vi "junk48.vi"() -> ()   [LabVIEW 2018]
uses:
  <vilib>/FTP/NI_FTP.lvlib
  <vilib>/Utility/error.llb/DialogType.ctl
panel:
  out "standard output":string
  out "message":string=" INSTRUCTIONS:\r\rNormal Use:  When using subVIs that incorporate the error in/error out (or error I/O) structure, place this handler where you want to inform the user of an error, typically at the end of the I/O data path, as the last action of the program.  If the error in error? is ERROR, the handler creates a message describing the error and its source.  If the type of dialog = 1 (default), the message is displayed to the user, who can only acknowedge it.  If the type = 2, the user can acknowledge the message or abort execution; aborting a program with active I/O is not recommended.  If the type = 0, no message is displayed; this is used to process the error programmatically, and the error out cluster elements are wired to individual terminals for that reason.  \r\rOther Use:\n\r\nlocal testing.  To test the error code of a subVI or function that does not have the error I/O structure, you can wire its error code and a source string to the local error code and error source inputs.  If error in error? indicates no error and error code is not equal to 0, the local code and source are substituted for the error in values, and error? is set TRUE (ERROR)."
  out "text 2":string
  in  "file (use dialog) 2":path=path "C:/tmp/junk1.txt"
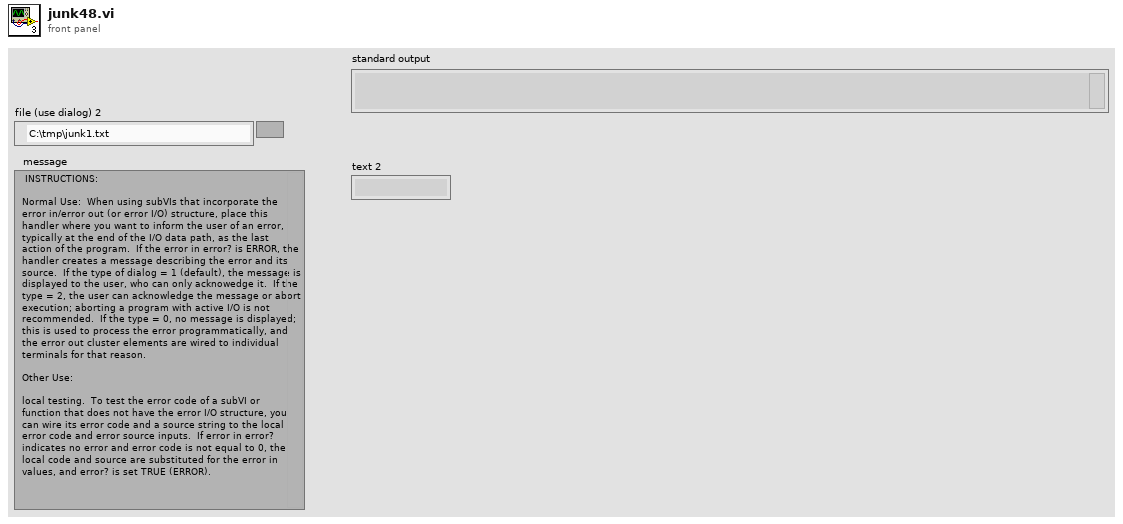
[diagram p1: front panel]
types:
  T1 = typedef "DialogType.ctl" = u16
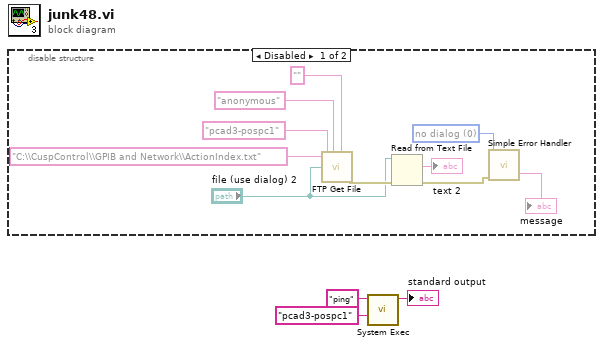
[diagram p0: block diagram]
diagram:
  n1 = disable-structure shown="Disabled" {
    frame Disabled {
      w5 = T1 0 items=["no dialog", "OK message", "continue or stop message", "OK message + warnings", "continue/stop + warnings"] ("type of dialog (OK msg:1)")
      n2 = call <vilib>:"FTP Get File.vi"("password"="", "user"="anonymous", "local path"="file (use dialog) 2", "remote path"="C:\\CuspControl\\GPIB and Network\\ActionIndex.txt", "host"="pcad3-pospc1") -> ("error out"=w9:errorcluster)  [unwired: 5 in, 1 out]
      n3 = Read from Text File(file (use dialog)="file (use dialog) 2", error in=w9) -> (text=→"text 2":string, error out=w6:errorcluster)  [unwired: 2 in, 2 out]
      n4 = call <vilib>:"Simple Error Handler.vi"("type of dialog (OK msg:1)"=w5, "error in (no error)"=w6) -> ("message"=→"message":string)  [unwired: 3 in, 4 out]
    }
    frame Enabled {
    }
  }
  n5 = call <vilib>:"System Exec.vi"("standard input"="pcad3-pospc1", "command line"="ping") -> ("standard output"=→"standard output":string)  [unwired: 6 in, 3 out]
